vi "Phasor Demo.vi"() -> ()   [LabVIEW 2016]
panel:
  out "Sample":bool
  out "Time [s]":dbl format="%.1f"
  out "Next sample [s]":dbl format="%.1f"
  in  "Update Interval [ms]":u32=100
  in  "fs [S/s]":dbl=1.0 min=1.0 max=1000.0 step=0.1 format="%#_13g"
  in  "Stop":bool
  in  "f [Hz]":dbl=1.0 format="%#_13g"
  out "XY Graph":cluster{dbl[], dbl[]}[](graph)
  # "Aliasing. Rotating phasor"
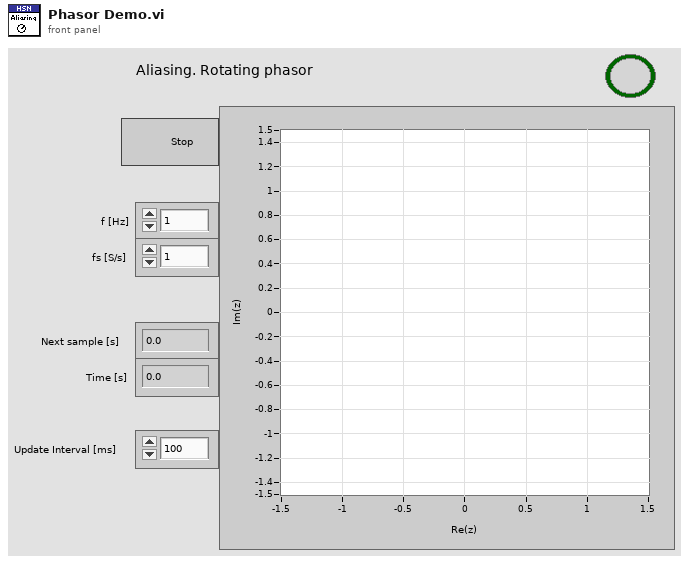
[diagram p1: front panel]
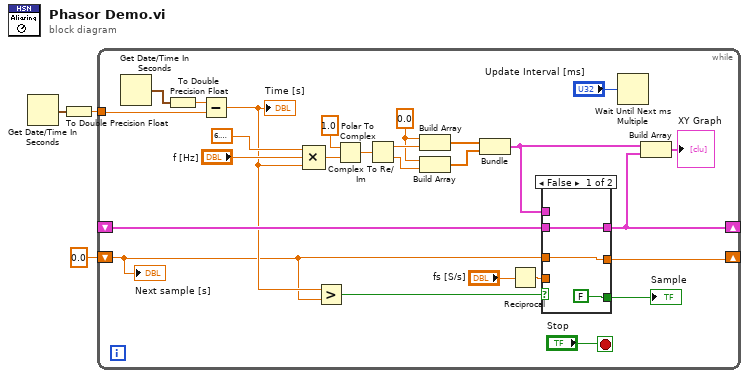
[diagram p0: block diagram]
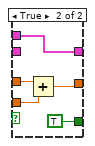
[diagram p2: hidden frame]
diagram:
  n1 = Get Date/Time In Seconds() -> (seconds since 1Jan1904=w2:timestamp)
  n2 = To Double Precision Float(number=w2) -> (double precision float=w1:dbl)
  n3 = while {
    shift-right: [w15] -> _
    shift-left: _ -> [w14]
    shift-right: [w12] -> _
    shift-left: 0.0 -> [w5]
    tunnel: w1 -> [w8]
    stop <- "Stop" stop-if-true
    w21 = 0.0 ("r")
    n4 = Get Date/Time In Seconds() -> (seconds since 1Jan1904=w9:timestamp)
    n5 = To Double Precision Float(number=w9) -> (double precision float=w7:dbl)
    n6 = Subtract(x=w7, y=w8) -> (x-y=w6:dbl)
    "Time [s]" <- w6
    n7 = Compound Arithmetic op=MULTIPLY(6.283185307179586, "f [Hz]", w6) -> (w28:dbl)
    n8 = Greater?(x=w6, y=w5) -> (0:w17:bool)
    n9 = Polar To Complex(1:w28, 2:1.0 ("r")) -> (0:w25:cdb)
    n10 = Complex To Re/Im(x + iy=w25) -> (x=w23:dbl, y=w22:dbl)
    n11 = Build Array(w21, w23) -> (w20:dbl[])
    n12 = Build Array(w21, w22) -> (w19:dbl[])
    n13 = Bundle(w20, w19) -> (w16:cluster{dbl[], dbl[]})  [unwired: 1 in]
    n14 = Reciprocal(x="fs [S/s]") -> (1/x=w13:dbl)
    n15 = case shown="False" w17 {
      tunnel: w16 -> [_ w37]
      tunnel: w5 -> [w32 w36]
      tunnel: [w32 w34] -> w12
      tunnel: [w31 w37] -> w15
      tunnel: w14 -> [w31 _]
      tunnel: w13 -> [_ w35]
      tunnel: [FALSE TRUE] -> w4
      frame False {
      }
      frame True {
        n16 = Add(x=w36, y=w35) -> (x+y=w34:dbl)
      }
    }
    "Sample" <- w4
    n17 = Wait Until Next ms Multiple(millisecond multiple="Update Interval [ms]") -> ()  [unwired: 1 out]
    n18 = Build Array(w16, w15) -> (→"XY Graph":cluster{dbl[], dbl[]}[])
    "Next sample [s]" <- w5
  }
